vi "FlatToRichni_protobuf_types_DoubleAnalogWaveform_AttributesEntry.vi"(5 "OutputClusterType":T1, 11 "InputCluster":T3) -> (3 "OutputCluster":T1)   [LabVIEW 2020, in "ni.protobuf.types.lvlib"]
uses:
  ni.protobuf.types.lvlib
  ni_protobuf_types_DoubleAnalogWaveform_AttributesEntry_Flat.ctl
  ni_protobuf_types_WaveformAttributeValue_Flat.ctl
  ni_protobuf_types_DoubleAnalogWaveform_AttributesEntry.ctl
  ni_protobuf_types_WaveformAttributeValue_attribute/ni_protobuf_types_WaveformAttributeValue_attribute.lvclass
  ni_protobuf_types_WaveformAttributeValue.ctl
  ni_protobuf_types_WaveformAttributeValue_attribute/ni_protobuf_types_WaveformAttributeValue_attribute.lvclass/ni_protobuf_types_WaveformAttributeValue_attribute.ctl
  ni_protobuf_types_WaveformAttributeValue_attribute/Setbool_value.vi
  ni_protobuf_types_WaveformAttributeValue_attribute/Setinteger_value.vi
  ni_protobuf_types_WaveformAttributeValue_attribute/Setdouble_value.vi
  ni_protobuf_types_WaveformAttributeValue_attribute/Setstring_value.vi
  ni_protobuf_types_WaveformAttributeValue_attribute/GetFieldFromProtobufIndexni_protobuf_types_WaveformAttributeValue_attribute.vi
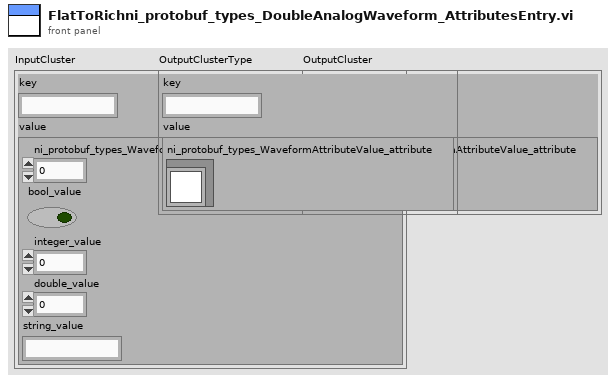
[diagram p1: front panel]
types:
  T1 = typedef "ni.protobuf.types.lvlib/ni_protobuf_types_DoubleAnalogWaveform_AttributesEntry.ctl" = cluster{"key":string, "value":T2}
  T2 = typedef "ni.protobuf.types.lvlib/ni_protobuf_types_WaveformAttributeValue.ctl" = cluster{"ni_protobuf_types_WaveformAttributeValue_attribute":refnum<class "ni_protobuf_types_WaveformAttributeValue_attribute.lvclass">}
  T3 = typedef "ni.protobuf.types.lvlib/ni_protobuf_types_DoubleAnalogWaveform_AttributesEntry_Flat.ctl" = cluster{"key":string, "value":T4}
  T4 = typedef "ni.protobuf.types.lvlib/ni_protobuf_types_WaveformAttributeValue_Flat.ctl" = cluster{"ni_protobuf_types_WaveformAttributeValue_attribute_selected_index":i32, "bool_value":bool, "integer_value":i32, "double_value":dbl, "string_value":string}
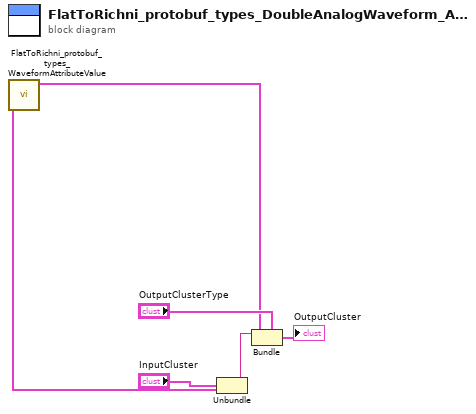
[diagram p0: block diagram]
diagram:
  n1 = Unbundle "Unbundle"("InputCluster") -> ("key"=w3:string, "value"=w2:T4)
  n2 = call "FlatToRichni_protobuf_types_WaveformAttributeValue.vi"("InputCluster"=w2) -> ("OutputCluster"=w1:T2)  [unwired: 10 in]
  n3 = Bundle "Bundle"(cluster="OutputClusterType", "key"=w3, "value"=w1) -> (→"OutputCluster":T1)
